vi "Steering Encoder Reader.vi"   [LabVIEW 2009]
uses:
  <vilib>/eio/EIONode/EIONode.xnode
  Motor Control Global.vi
  <vilib>/rvi/eio/nirviEIOImplementation/nirviEIOImplementation.xnode
  <vilib>/rvi/eio/common/nirviEmuTemplateMethod_noerrors.vi
  <vilib>/rvi/eio/common/nirviEmuClasses.ctl
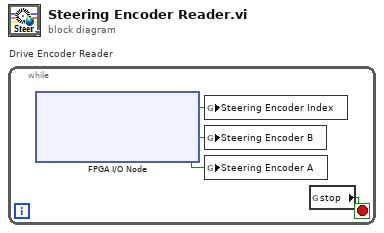
[diagram p0: block diagram]
diagram:
  n1 = while "Drive Encoder Reader" {
    stop <- w1 stop-if-true
    n2 = xnode "FPGA I/O Node"() -> ("Steering Encoder Index"=w4:bool, "Steering Encoder B"=w3:bool, "Steering Encoder A"=w2:bool)  [unwired: 3 in, 3 out]
    n3 = global write "Motor Control Global.vi" "Steering Encoder Index"(w4) -> ()
    n4 = global write "Motor Control Global.vi" "Steering Encoder B"(w3) -> ()
    n5 = global write "Motor Control Global.vi" "Steering Encoder A"(w2) -> ()
    n6 = global read "Motor Control Global.vi" "stop"() -> (w1:bool)
  }
